vi "DeleteLayer.vi"(6 "error in":errorcluster, 7 "AntsRect":T8, 9 "Data in":T1={"Class"={"Ants"=refnum, "Layer"=refnum, "Templates"=refnum, "Icon"=refnum, "Glyph"=refnum, "Settings"=refnum, "Tools"=refnum}, "Ref"={"Add Layer"=refnum, "Remove Layer"=refnum, "Line Text"=[], "Body Text Spec"=refnum, "DNL_Font"=refnum, "glyph path str"=refnum, "templates path str"=refnum, "Arrow Up"=refnum, "Arrow Down"=refnum, "IE VI Ref"=refnum, "Glyphs tree"=refnum, "Templates tree"=refnum, "Layer Icon Text"=refnum, "Layer Template"=refnum, "Body Text"=refnum, "Search Templates"=refnum, "TextMarker"=refnum, "Tab Control"=refnum, "Search Glyphs"=refnum, "Line Color"=refnum, "DNL_Glyphs []"=refnum, "Fill Color"=refnum, "Tools"=refnum, "Icon"=refnum, "Preview"=refnum, "Ants"=refnum, "Terminals"=refnum, "menu reference"=refnum, "LayerNames"=[], "GlyphLoadAnimation"=refnum, "TemplateLoadAnimation"=refnum, "refreshGlyphs"=refnum, "refreshTemplates"=refnum}, "Support"={"AntsRect"={"left"=0, "top"=0, "right"=0, "bottom"=0}, "Mouse Move Coords"={"Horizontal"=0, "Vertical"=0}, "Mouse Down Coords"={"Horizontal"=0, "Vertical"=0}, "Temp Coord"={"Horizontal"=0, "Vertical"=0}, "Action"=enum."Default", "Edge Color"=4914962, "Fill Color"=16860, "Mouse Down?"=FALSE, "Draft Mode?"=FALSE, "Temp Icon"=bytes[3102], "CTRL Pressed"=FALSE, "Move Selection?"=FALSE, "AntsRect Orig"={"left"=0, "top"=0, "right"=0, "bottom"=0}, "Text"="", "TM Set?"=FALSE, "Mouse inside icon?"=FALSE, "Tool (old value)"=0, "Pencil Move Color"=0, "Swap Colors?"=FALSE, "Shift pressed?"=FALSE}}) -> (0 "error out":errorcluster, 3 "Data out":T1={"Class"={"Ants"=refnum, "Layer"=refnum, "Templates"=refnum, "Icon"=refnum, "Glyph"=refnum, "Settings"=refnum, "Tools"=refnum}, "Ref"={"Add Layer"=refnum, "Remove Layer"=refnum, "Line Text"=[], "Body Text Spec"=refnum, "DNL_Font"=refnum, "glyph path str"=refnum, "templates path str"=refnum, "Arrow Up"=refnum, "Arrow Down"=refnum, "IE VI Ref"=refnum, "Glyphs tree"=refnum, "Templates tree"=refnum, "Layer Icon Text"=refnum, "Layer Template"=refnum, "Body Text"=refnum, "Search Templates"=refnum, "TextMarker"=refnum, "Tab Control"=refnum, "Search Glyphs"=refnum, "Line Color"=refnum, "DNL_Glyphs []"=refnum, "Fill Color"=refnum, "Tools"=refnum, "Icon"=refnum, "Preview"=refnum, "Ants"=refnum, "Terminals"=refnum, "menu reference"=refnum, "LayerNames"=[], "GlyphLoadAnimation"=refnum, "TemplateLoadAnimation"=refnum, "refreshGlyphs"=refnum, "refreshTemplates"=refnum}, "Support"={"AntsRect"={"left"=0, "top"=0, "right"=0, "bottom"=0}, "Mouse Move Coords"={"Horizontal"=0, "Vertical"=0}, "Mouse Down Coords"={"Horizontal"=0, "Vertical"=0}, "Temp Coord"={"Horizontal"=0, "Vertical"=0}, "Action"=enum."Default", "Edge Color"=4914962, "Fill Color"=16860, "Mouse Down?"=FALSE, "Draft Mode?"=FALSE, "Temp Icon"=bytes[3102], "CTRL Pressed"=FALSE, "Move Selection?"=FALSE, "AntsRect Orig"={"left"=0, "top"=0, "right"=0, "bottom"=0}, "Text"="", "TM Set?"=FALSE, "Mouse inside icon?"=FALSE, "Tool (old value)"=0, "Pencil Move Color"=0, "Swap Colors?"=FALSE, "Shift pressed?"=FALSE}})   [LabVIEW 2021]
uses:
  <resource>/plugins/NIIconEditor/Class/Ants/Ants.lvclass
  <resource>/plugins/NIIconEditor/Class/FakedArray/FakedArray.lvclass
  <vilib>/LabVIEW Icon API/lv_icon/Classes/Icon/Icon.lvclass
  <resource>/plugins/NIIconEditor/Class/Icon Library/Glyph.lvclass
  <resource>/plugins/NIIconEditor/Class/Settings/Settings.lvclass
  <resource>/plugins/NIIconEditor/Class/Tools/Tools Paint.lvclass
  <vilib>/LabVIEW Icon API/lv_icon/Classes/Layer/Layer.lvclass
  <vilib>/LabVIEW Icon API/lv_icon/lv_icon.lvlib
  <vilib>/Utility/miscctls.llb/LVPoint32TypeDef.ctl
  <resource>/plugins/NIIconEditor/Controls/SupportClass_Action.ctl
  <vilib>/LabVIEW Icon API/lv_icon/Controls/IEColor.ctl
  <resource>/plugins/NIIconEditor/Controls/SupportClass.ctl
  <resource>/plugins/NIIconEditor/Controls/References Cluster.ctl
  <resource>/plugins/NIIconEditor/Controls/IE Classes.ctl
  <resource>/plugins/NIIconEditor/Controls/Global Data.ctl
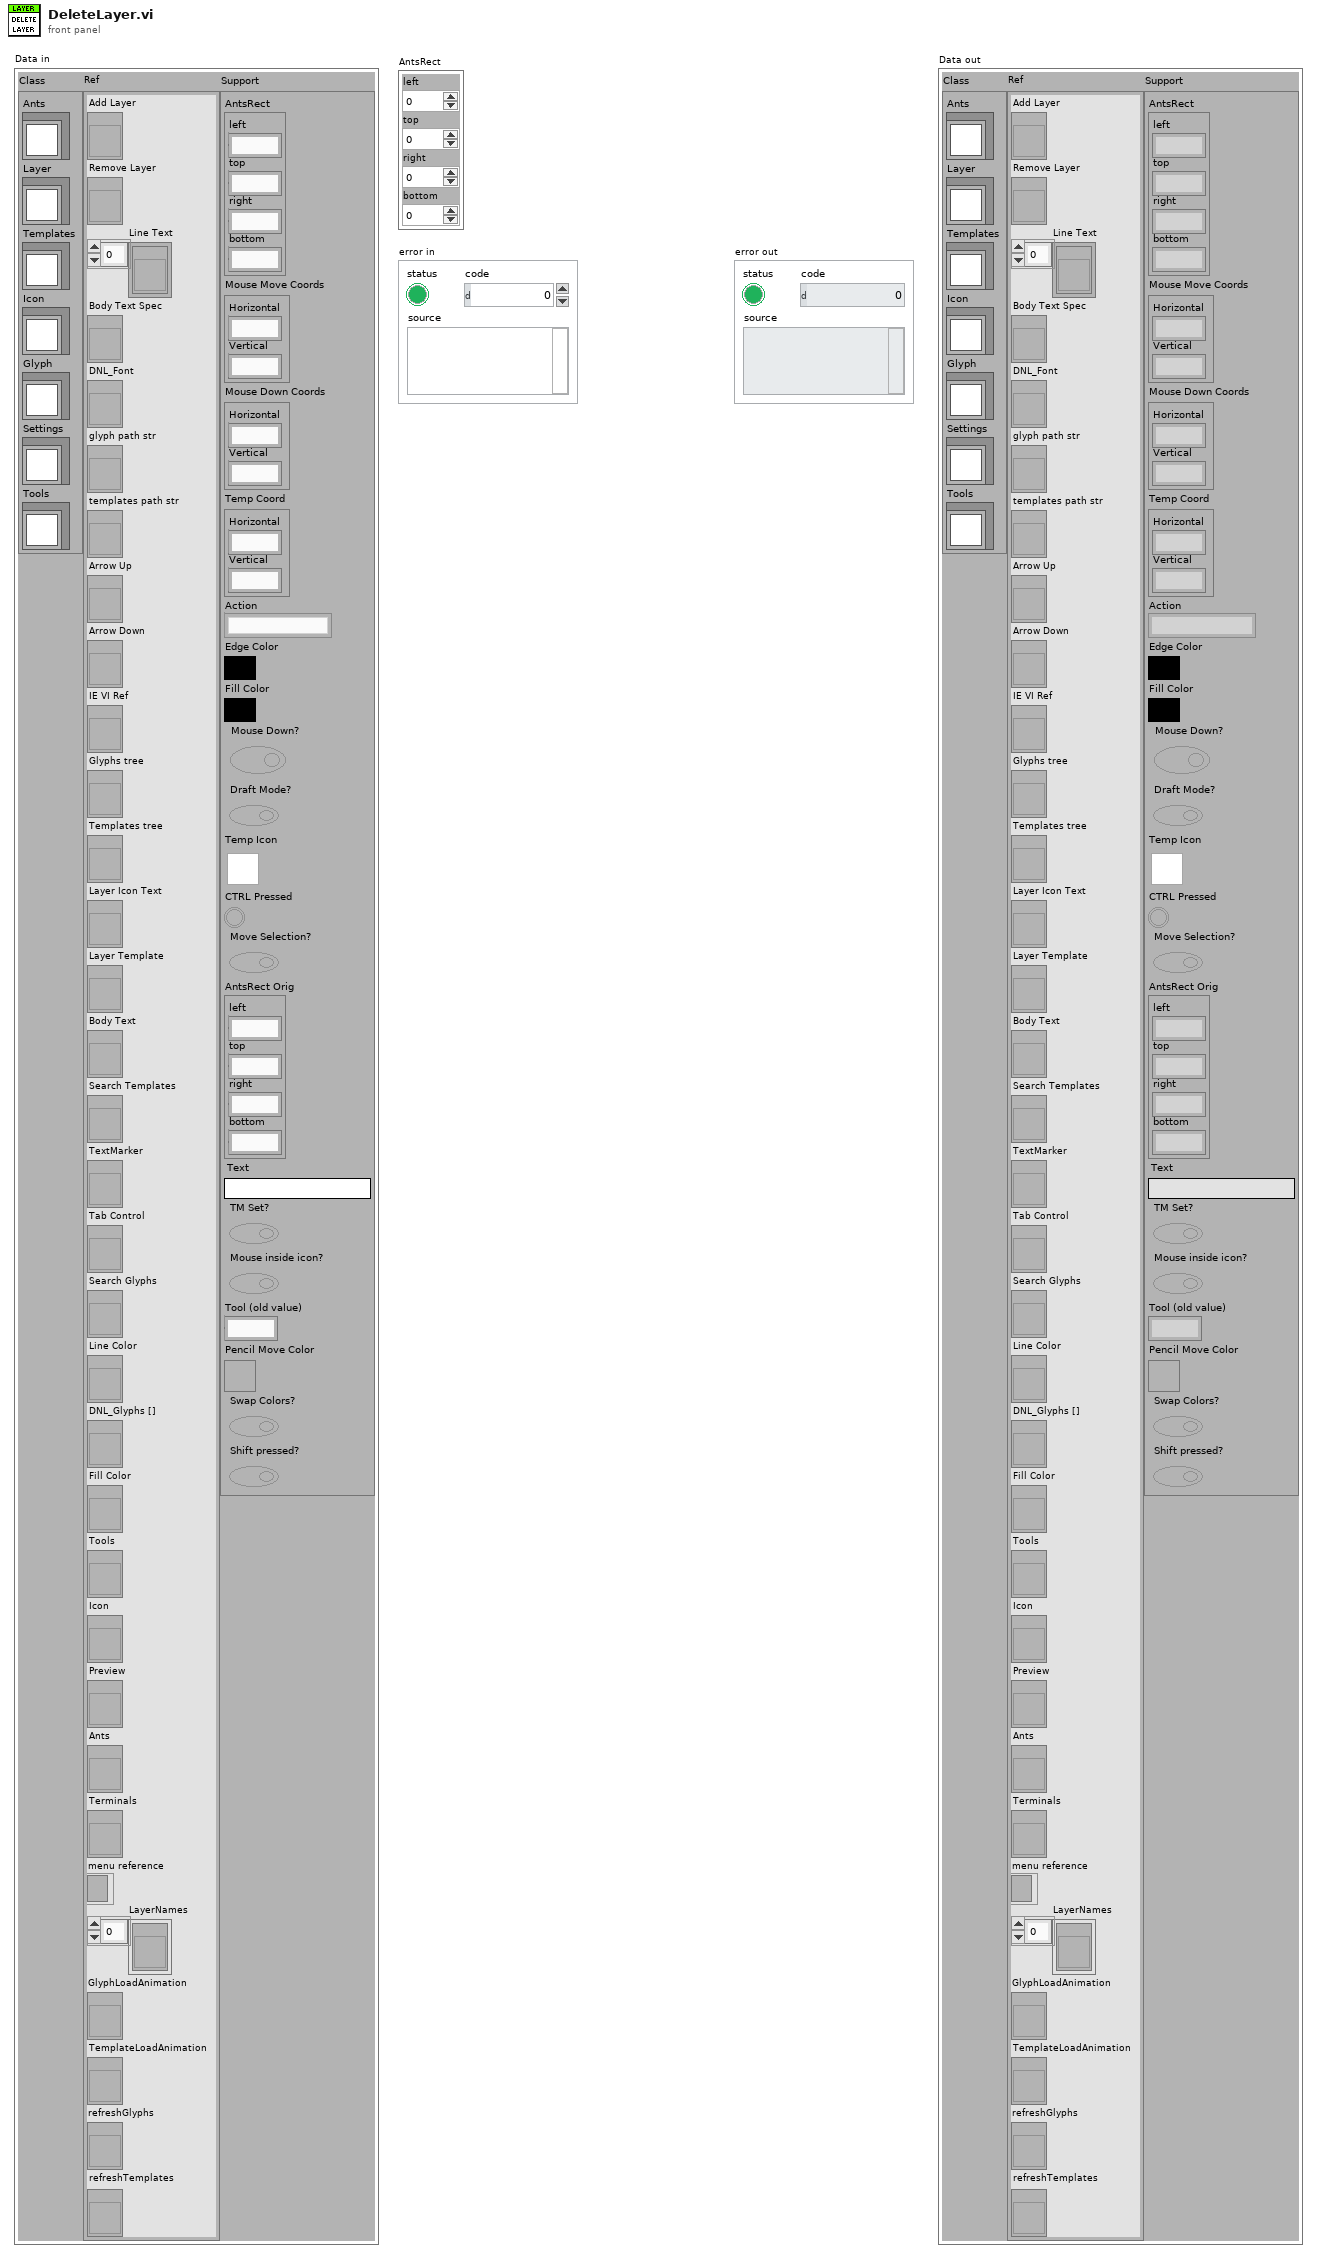
[diagram p1: front panel]
types:
  T1 = typedef "lv_icon.lvlib/Global Data.ctl" = cluster{"Class":T2, "Ref":T3, "Support":T4}
  T2 = typedef "IE Classes.ctl" = cluster{"Ants":refnum<class "Ants.lvclass">, "Layer":refnum<class "FakedArray.lvclass">, "Templates":refnum<class "FakedArray.lvclass">, "Icon":refnum<class "Icon.lvclass">, "Glyph":refnum<class "Glyph.lvclass">, "Settings":refnum<class "Settings.lvclass">, "Tools":refnum<class "Tools Paint.lvclass">}
  T3 = typedef "lv_icon.lvlib/References Cluster.ctl" = cluster{"Add Layer":refnum<vi>, "Remove Layer":refnum<vi>, "Line Text":refnum<vi>[], "Body Text Spec":refnum<vi>, "DNL_Font":refnum<vi>, "glyph path str":refnum<vi>, "templates path str":refnum<vi>, "Arrow Up":refnum<vi>, "Arrow Down":refnum<vi>, "IE VI Ref":refnum<vi>, "Glyphs tree":refnum<vi>, "Templates tree":refnum<vi>, "Layer Icon Text":refnum<vi>, "Layer Template":refnum<vi>, "Body Text":refnum<vi>, "Search Templates":refnum<vi>, "TextMarker":refnum<vi>, "Tab Control":refnum<vi>, "Search Glyphs":refnum<vi>, "Line Color":refnum<vi>, "DNL_Glyphs []":refnum<vi>, "Fill Color":refnum<vi>, "Tools":refnum<vi>, "Icon":refnum<vi>, "Preview":refnum<vi>, "Ants":refnum<vi>, "Terminals":refnum<vi>, "menu reference":refnum<k9>, "LayerNames":refnum<vi>[], "GlyphLoadAnimation":refnum<vi>, "TemplateLoadAnimation":refnum<vi>, "refreshGlyphs":refnum<vi>, "refreshTemplates":refnum<vi>}
  T4 = typedef "SupportClass.ctl" = cluster{"AntsRect":cluster{"left":i16, "top":i16, "right":i16, "bottom":i16}, "Mouse Move Coords":T5, "Mouse Down Coords":T5, "Temp Coord":T5, "Action":T6, "Edge Color":T7, "Fill Color":T7, "Mouse Down?":bool, "Draft Mode?":bool, "Temp Icon":picture, "CTRL Pressed":bool, "Move Selection?":bool, "AntsRect Orig":cluster{"left":i16, "top":i16, "right":i16, "bottom":i16}, "Text":string, "TM Set?":bool, "Mouse inside icon?":bool, "Tool (old value)":u32, "Pencil Move Color":u32, "Swap Colors?":bool, "Shift pressed?":bool}
  T5 = typedef "LVPoint32TypeDef.ctl" = cluster{"Horizontal":i32, "Vertical":i32}
  T6 = typedef "SupportClass_Action.ctl" = enum16{"Default", "Move Selection", "Glyph Library", "Tool"}
  T7 = typedef "IEColor.ctl" = u32
  T8 = cluster{"left":i16, "top":i16, "right":i16, "bottom":i16}
  T9 = typedef "Layer.ctl" = cluster{"LayerIcon":picture, "LayerName":string, "Opacity":u8, "Visibility?":bool}
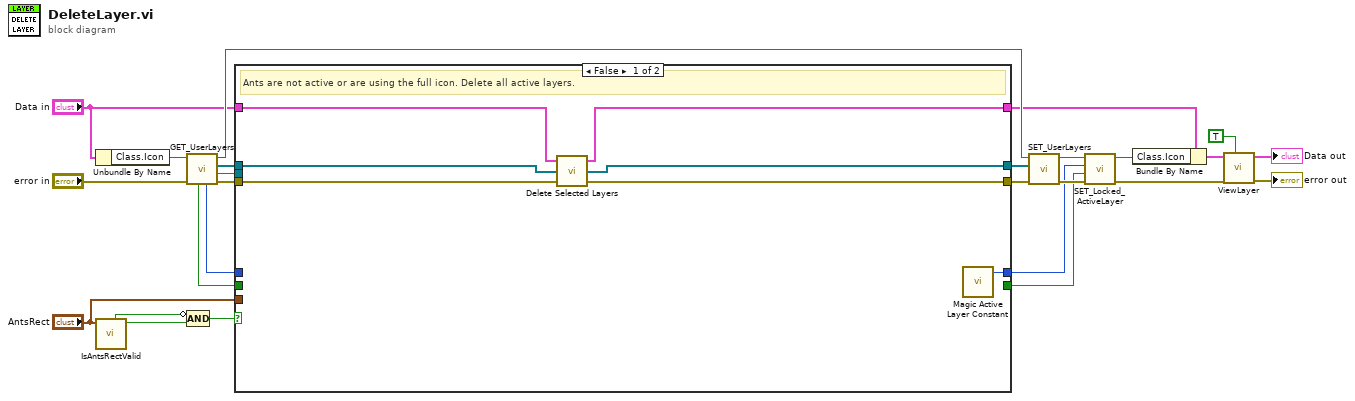
[diagram p0: block diagram]
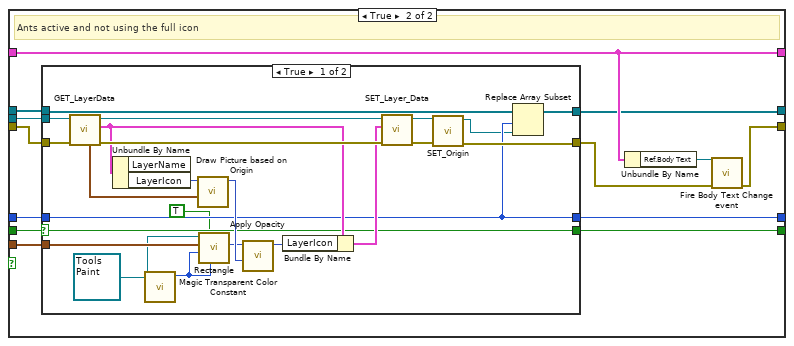
[diagram p2: hidden frame]
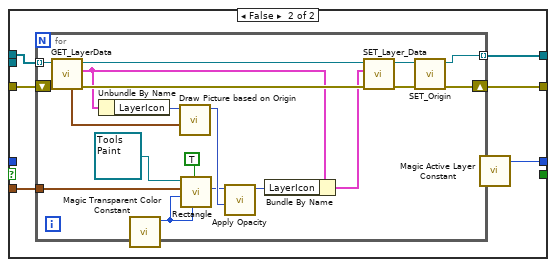
[diagram p3: hidden frame]
diagram:
  n1 = Unbundle By Name("Data in") -> ("Class.Icon"=w12:refnum<class "Icon.lvclass">)
  n2 = call <resource>:"IsAntsRectValid.vi"("AntsRect"="AntsRect") -> ("Valid?"=w3:bool, "Max. Rect size?"=w2:bool)  [unwired: 9 out]
  n3 = call-dynamic "GET_UserLayers.vi"("error in (no error)"="error in", "Icon.lvclass in"=w12) -> ("error out"=w25:errorcluster, "Active Layer"=w17:refnum<class "Layer.lvclass">, "All Layers"=w18:refnum<class "Layer.lvclass">[], "Icon.lvclass out"=w20:refnum<class "Icon.lvclass">, "#Active Layer"=w19:i32, "Layer Locked?"=w16:bool)  [unwired: 4 out]
  n4 = Compound Arithmetic op=AND(invert w2, w3) -> (w1:bool)
  n5 = case shown="False" w1 {
    tunnel: [w33 w44] -> w26
    tunnel: [w31 w37] -> w4
    tunnel: w19 -> [_ w41]
    tunnel: w25 -> [w32 w46]
    tunnel: w18 -> [w30 w38]
    tunnel: w17 -> [_ w40]
    tunnel: w16 -> [_ w42]
    tunnel: "AntsRect" -> [_ w39]
    tunnel: [w29 w36] -> w14
    tunnel: [_ w35] -> w13
    tunnel: "Data in" -> [w28 w43]
    tunnel: [w27 w43] -> w9
    frame False {
      # "Ants are not active or are using the full icon. Delete all active layers."
      n6 = call <resource>:"Delete Selected Layers.vi"("error in"=w32, "All Layers in"=w30, "Data in"=w28) -> ("error out"=w33:errorcluster, "All Layers out"=w31:refnum<class "Layer.lvclass">[], "Data out"=w27:T1)
      n7 = call <resource>:"Magic Active Layer Constant.vi"() -> ("Magic Constant"=w29:i32)  [unwired: 19 out]
    }
    frame True {
      # "Ants active and not using the full icon"
      n8 = case shown="True" w42 {
        selector: w42 -> [w52 _]
        tunnel: w41 -> [w53 _]
        tunnel: w40 -> [w65 _]
        tunnel: w46 -> [w69 w75]
        tunnel: w39 -> [w62 w73]
        tunnel: [w67 w74] -> w45
        tunnel: w38 -> [w55 w72]
        tunnel: [w54 w71] -> w37
        tunnel: [w53 w70] -> w36
        tunnel: [w52 _] -> w35
        frame True {
          n9 = call-dynamic "GET_LayerData.vi"("error in (no error)"=w69, "Layer.lvclass in"=w65) -> ("error out"=w66:errorcluster, "Data"=w59:T9, "Layer.lvclass out"=w57:refnum<class "Layer.lvclass">, "Origin"=w63:T5)  [unwired: 6 out]
          n10 = Unbundle By Name(w59) -> ("LayerIcon"=w64:picture)  [unwired: 1 out]
          n11 = call <vilib>:"Magic Transparent Color Constant.vi"() -> ("Magic transparent color constant"=w49:u32)  [unwired: 11 out]
          n12 = call <vilib>:"Draw Picture based on Origin.vi"("Origin"=w63, "LayerIcon in"=w64) -> ("LayerIcon out"=w61:picture)  [unwired: 1 in, 8 out]
          n13 = call-dynamic "Rectangle.vi"("Fill Color"=w49, "fill?(F)"=TRUE, "Edge Color"=w49, "rect"=w62, "Tools Paint in"=refnum<class "Tools Paint.lvclass"> refnum) -> ("new picture"=w60:picture)  [unwired: 1 in, 5 out]
          n14 = call <vilib>:"Apply Opacity.vi"("Bottom"=w61, "Top"=w60) -> ("new picture"=w58:picture)  [unwired: 1 in, 8 out]
          n15 = Bundle By Name(cluster=w59, "LayerIcon"=w58) -> (w56:T9)
          n16 = call-dynamic "SET_Layer_Data.vi"("error in (no error)"=w66, "Data"=w56, "Layer.lvclass in"=w57) -> ("error out"=w68:errorcluster, "Layer.lvclass out"=w48:refnum<class "Layer.lvclass">)  [unwired: 1 in, 6 out]
          n17 = call-dynamic "SET_Origin.vi"("error in"=w68, "Layer.lvclass in"=w48) -> ("error out"=w67:errorcluster, "Layer.lvclass out"=w47:refnum<class "Layer.lvclass">)  [unwired: 8 in]
          n18 = Replace Array Subset(array=w55, new element=w47, index=w53) -> (w54:refnum<class "Layer.lvclass">[])
        }
        frame False {
          n19 = for {
            tunnel: w73 -> [w88]
            shift-right: [w92] -> w74
            shift-left: w75 -> [w94]
            tunnel: w72 -> [w81] mode=indexing
            tunnel: [w76] -> w71 mode=indexing
            n20 = call-dynamic "GET_LayerData.vi"("error in (no error)"=w94, "Layer.lvclass in"=w81) -> ("error out"=w91:errorcluster, "Data"=w85:T9, "Layer.lvclass out"=w83:refnum<class "Layer.lvclass">, "Origin"=w89:T5)  [unwired: 6 out]
            n21 = Unbundle By Name(w85) -> ("LayerIcon"=w90:picture)
            n22 = call <vilib>:"Magic Transparent Color Constant.vi"() -> ("Magic transparent color constant"=w78:u32)  [unwired: 11 out]
            n23 = call <vilib>:"Draw Picture based on Origin.vi"("Origin"=w89, "LayerIcon in"=w90) -> ("LayerIcon out"=w87:picture)  [unwired: 1 in, 8 out]
            n24 = call-dynamic "Rectangle.vi"("Fill Color"=w78, "fill?(F)"=TRUE, "Edge Color"=w78, "rect"=w88, "Tools Paint in"=refnum<class "Tools Paint.lvclass"> refnum) -> ("new picture"=w86:picture)  [unwired: 1 in, 5 out]
            n25 = call <vilib>:"Apply Opacity.vi"("Bottom"=w87, "Top"=w86) -> ("new picture"=w84:picture)  [unwired: 1 in, 8 out]
            n26 = Bundle By Name(cluster=w85, "LayerIcon"=w84) -> (w82:T9)
            n27 = call-dynamic "SET_Layer_Data.vi"("error in (no error)"=w91, "Data"=w82, "Layer.lvclass in"=w83) -> ("error out"=w93:errorcluster, "Layer.lvclass out"=w77:refnum<class "Layer.lvclass">)  [unwired: 1 in, 6 out]
            n28 = call-dynamic "SET_Origin.vi"("error in"=w93, "Layer.lvclass in"=w77) -> ("error out"=w92:errorcluster, "Layer.lvclass out"=w76:refnum<class "Layer.lvclass">)  [unwired: 8 in]
          }
          n29 = call <resource>:"Magic Active Layer Constant.vi"() -> ("Magic Constant"=w70:i32)  [unwired: 19 out]
        }
      }
      n30 = Unbundle By Name(w43) -> ("Ref.Body Text"=w34:refnum<vi>)
      n31 = call <resource>:"Fire Body Text Change event.vi"("error in"=w45, "Ref.Body Text"=w34) -> ("error out"=w44:errorcluster)  [unwired: 2 in, 7 out]
    }
  }
  n32 = call-dynamic "SET_UserLayers.vi"("error in (no error)"=w26, "Layers"=w4, "Icon.lvclass in"=w20) -> ("error out"=w24:errorcluster, "Icon.lvclass out"=w7:refnum<class "Icon.lvclass">)  [unwired: 7 in]
  n33 = call-dynamic "SET_Locked_ActiveLayer.vi"("error in (no error)"=w24, "Layers Locked?"=w13, "Active Layer"=w14, "Icon.lvclass in"=w7) -> ("error out"=w23:errorcluster, "Icon.lvclass out"=w10:refnum<class "Icon.lvclass">)  [unwired: 6 out]
  n34 = Bundle By Name(cluster=w9, "Class.Icon"=w10) -> (w6:T1)
  n35 = call <resource>:"ViewLayer.vi"("Add to Undo?"=TRUE, "error in (no error)"=w23, "Data in"=w6) -> ("error out"=→"error out":errorcluster, "Data out"=→"Data out":T1)  [unwired: 1 in, 6 out]
